vi "Test Data Acq.vi"() -> ()   [LabVIEW 2025]
doc: "Author: Scott Hannahs <sth@magnet.fsu.edu>\n\nThis software is licensed for use under the “MIT License\"\nCopyright (c) 2025 Scott Hannahs, sth@sth@magnet.sthnet.net\n\nPermission is hereby granted, free of charge, to any person obtaining a copy of this software and associated documentation files (the \"Software\"), to deal in the Software without restriction, including without limitation the rights to use, copy, modify, merge, publish, distribute, sublicense, and/or sell copies of the Software, and to permit persons to whom the Software is furnished to do so, subject to the following conditions: The above copyright notice and this permission notice shall be included in all copies or substantial portions of the Software.\n\nTHE SOFTWARE IS PROVIDED \"AS IS\", WITHOUT WARRANTY OF ANY KIND, EXPRESS OR IMPLIED, INCLUDING BUT NOT LIMITED TO THE WARRANTIES OF MERCHANTABILITY, FITNESS FOR A PARTICULAR PURPOSE AND NONINFRINGEMENT. IN NO EVENT SHALL THE AUTHORS OR COPYRIGHT HOLDERS BE LIABLE FOR ANY CLAIM, DAMAGES OR OTHER LIABILITY, WHETHER IN AN ACTION OF CONTRACT, TORT OR OTHERWISE, ARISING FROM, OUT OF OR IN CONNECTION WITH THE SOFTWARE OR THE USE OR OTHER DEALINGS IN THE SOFTWARE."
uses:
  Sub Controls/All Data Array.ctl
  Sub Controls/Instrument Properties.ctl
  Sub Controls/Public.ctl
  Sub Controls/Private.ctl
  Sub Controls/Instrument Ref.ctl
  Sub Controls/SystemCheckBox-resize.ctl
  Sub Controls/DataAcq User Events.ctl
panel:
  in  "New/Stop":bool
  out "All Data":T1 format="%^_6g"
  out "Labels":string[](array[string])=["Field", "Timestamp"]
  out "Data":dbl[](array[numeric])=[1.0, 0.02, 0.0, 0.0] format="%_4e"
  out "Colors":u32[](array[colorbox])=[16748168, 2796287]
  in  "Quit":bool
  in  "Test":bool
  in  "Configure":bool
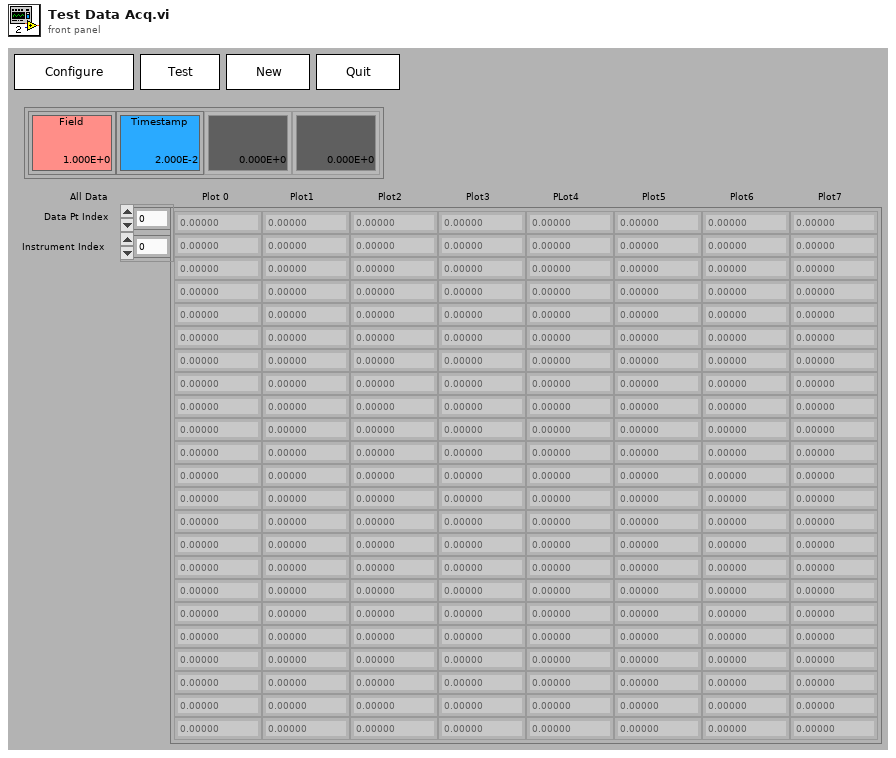
[diagram p1: front panel]
types:
  T1 = typedef "All Data Array.ctl" = dbl[][]
  T2 = typedef "DataAcq User Events.ctl" = enum16{"Update Data Display", "Store Data"}
  T3 = typedef "Instrument Properties.ctl" = cluster{"Public":T4, "Private":T5}
  T4 = typedef "Public.ctl" = cluster{"Column Name":string[], "Trace Color":u32[]}
  T5 = typedef "Private.ctl" = cluster{"Path":path, "VI Refnum":T6, "Name":string, "# of Values":i32, "Scale Factors":dbl[], "Display":T7[], "Offset":dbl[]}
  T6 = typedef "Instrument Ref.ctl" = refnum<vi>
  T7 = typedef "SystemCheckBox-resize.ctl" = bool
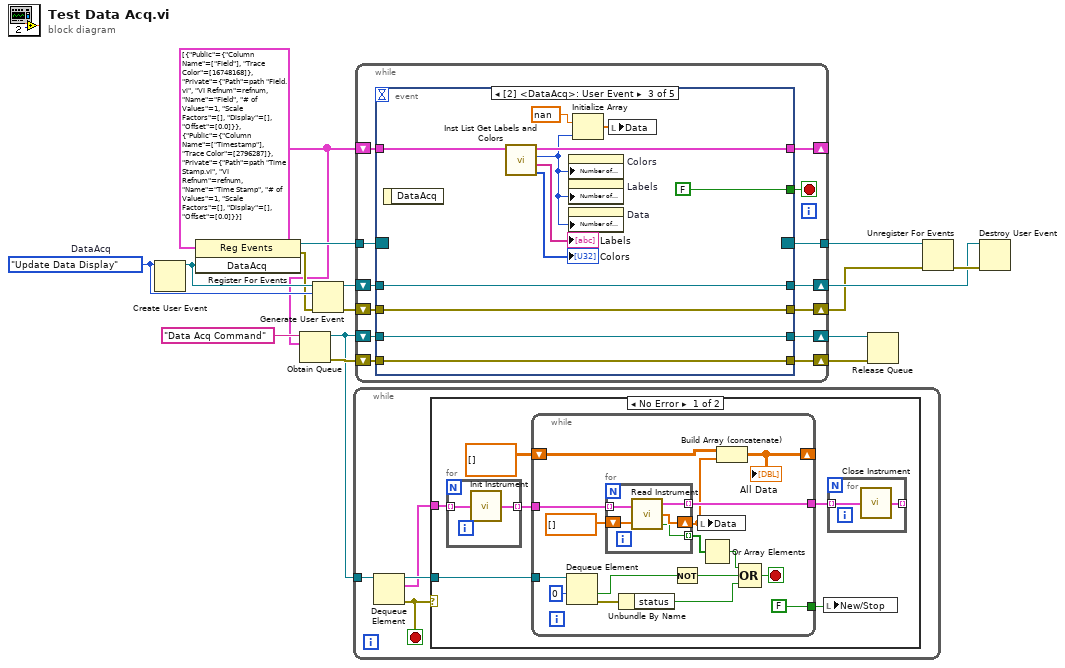
[diagram p0: block diagram]
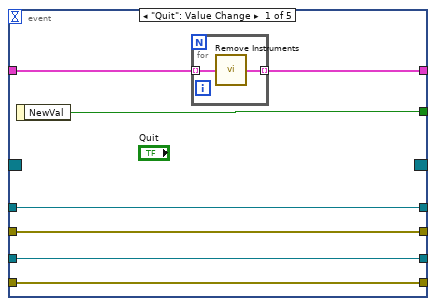
[diagram p3: hidden frame]
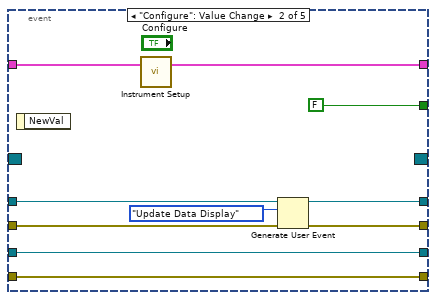
[diagram p4: hidden frame]
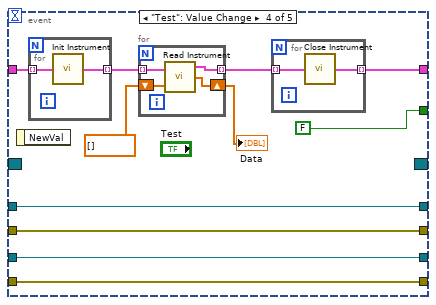
[diagram p5: hidden frame]
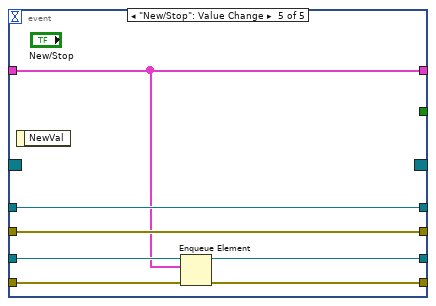
[diagram p6: hidden frame]
diagram:
  w14 = DataAcq_User_Events."Update Data Display"  # DataAcq
  w1 = T3[] [{"Public"={"Column Name"=["Field"], "Trace Color"=[16748168]}, "Private"={"Path"=path "Field.vi", "VI Refnum"=refnum, "Name"="Field", "# of Values"=1, "Scale Factors"=[], "Display"=[], "Offset"=[0.0]}}, {"Public"={"Column Name"=["Timestamp"], "Trace Color"=[2796287]}, "Private"={"Path"=path "Time Stamp.vi", "VI Refnum"=refnum, "Name"="Time Stamp", "# of Values"=1, "Scale Factors"=[], "Display"=[], "Offset"=[0.0]}}] ("Setup")
  n1 = Create User Event(user event datatype=w14) -> (user event=w15:refnum<user-event>)  [unwired: 1 in, 1 out]
  n2 = register-events(w15) -> (reference out=w16:refnum<event-registration>, error out=w13:errorcluster)  [unwired: 2 in]
  n3 = Obtain Queue(name (unnamed)="Data Acq Command", element data type=w1) -> (queue out=w3:refnum<queue>, error out=w5:errorcluster)  [unwired: 3 in, 1 out]
  n4 = Generate User Event(user event=w15, event data cluster=w14, error in=w13) -> (user event out=w12:refnum<user-event>, error out=w7:errorcluster)  [unwired: 1 in]
  n5 = while {
    tunnel: w3 -> [w20]
    stop <- w19 stop-if-true
    n6 = Dequeue Element(queue=w20) -> (queue out=w18:refnum<queue>, element=w17:T3[], error out=w19:errorcluster)  [unwired: 2 in, 1 out]
    n7 = case shown="No Error" w19 {
      tunnel: w18 -> [w22 _]
      tunnel: w17 -> [w26 _]
      frame No Error {
        n8 = for {
          tunnel: w26 -> [w51] mode=indexing
          tunnel: [w50] -> w25 mode=indexing
          n9 = call "Init Instrument.vi"("Instrument Prop"=w51) -> ("Instrument Prop 2"=w50:T3)
        }
        n10 = while {
          tunnel: w25 -> [w43]
          tunnel: [w42] -> w24
          shift-right: [w38] -> _
          shift-left: dbl[][] [] ("Array 2") -> [w37]
          tunnel: w22 -> [w34]
          tunnel: [FALSE ("New/Stop")] -> w21
          stop <- w39 stop-if-true
          n11 = Dequeue Element(queue=w34, timeout in ms (-1)=0) -> (timed out?=w35:bool, error out=w31:errorcluster)  [unwired: 1 in, 2 out]
          n12 = for {
            tunnel: w43 -> [w49] mode=indexing
            tunnel: [w48] -> w42 mode=indexing
            shift-right: [w46] -> w36
            shift-left: dbl[] [] ("Array 2") -> [w47]
            tunnel: [w45] -> w41 mode=indexing
            n13 = call "Read Instrument.vi"("Instrument Prop In"=w49, "Array In"=w47) -> ("Instrument Prop Out"=w48:T3, "Array Out"=w46:dbl[], "Stop"=w45:bool)
          }
          n14 = Unbundle By Name(w31) -> ("status"=w32:bool)
          n15 = Not(x=w35) -> (.not. x?=w30:bool)
          n16 = local write "Data"(w36) -> ()
          n17 = Or Array Elements(Boolean array=w41) -> (logical OR=w40:bool)
          n18 = Build Array (concatenate)(w37, w36) -> (w38:dbl[][])
          "All Data" <- w38
          n19 = Compound Arithmetic op=OR(w40, w30, w32) -> (w39:bool)
        }
        n20 = local write "New/Stop"(w21) -> ()
        n21 = for {
          tunnel: w24 -> [w28] mode=indexing
          tunnel: [w27] -> _ mode=indexing
          n22 = call "Close Instrument.vi"("Instrument Prop"=w28) -> ("Instrument Prop 2"=w27:T3)
        }
      }
      frame Error {
      }
    }
  }
  n23 = while {
    shift-right: [w63] -> _
    shift-left: w1 -> [w62]
    tunnel: w16 -> [w61]
    shift-right: [w59] -> w9
    shift-left: w12 -> [w60]
    tunnel: [w58] -> w11
    shift-right: [w56] -> w8
    shift-left: w3 -> [w57]
    shift-right: [w54] -> w6
    shift-left: w7 -> [w55]
    shift-right: [w52] -> w4
    shift-left: w5 -> [w53]
    stop <- w64 stop-if-true
    n24 = event shown="[2] <DataAcq>: User Event" {
      selector: w61 -> [_ _ _ _ _]
      dyn-events: [_ _ _ _ _] -> w58
      timeout: _ -> [_ _ _ _ _]
      tunnel: [w69 FALSE ("stop") FALSE ("stop") FALSE ("stop") _] -> w64
      tunnel: w62 -> [w71 w83 w93 w101 w115]
      tunnel: [w70 w78 w94 w99 w115] -> w63
      tunnel: w60 -> [w68 w81 w90 w103 w121]
      tunnel: [w68 w79 w90 w103 w121] -> w59
      tunnel: [w66 w75 w85 w98 w119] -> w56
      tunnel: w57 -> [w66 w75 w85 w98 w116]
      tunnel: [w67 w77 w86 w97 w120] -> w54
      tunnel: w55 -> [w67 w76 w86 w97 w120]
      tunnel: [w65 w74 w84 w96 w118] -> w52
      tunnel: w53 -> [w65 w74 w84 w96 w117]
      event "Quit": Value Change {
        n25 = event-data() -> ("NewVal"=w69:bool)  [unwired: 1 in]
        n26 = for {
          tunnel: w71 -> [w73] mode=indexing
          tunnel: [w72] -> w70 mode=indexing
          n27 = call "Remove Instruments.vi"("Instrument Prop"=w73) -> ("Instrument Prop Out"=w72:T3)
        }
      }
      event "Configure": Value Change {
        n28 = event-data() -> ()  [unwired: 1 in, 1 out]
        n29 = call "Instrument Setup.vi"("Configured Inst"=w83) -> ("Configured Inst dup"=w78:T3[])  [unwired: 2 in]
        n30 = Generate User Event(user event=w81, event data cluster=DataAcq_User_Events."Update Data Display" ("event data"), error in=w76) -> (user event out=w79:refnum<user-event>, error out=w77:errorcluster)  [unwired: 1 in]
      }
      event User Event {
        n31 = event-data() -> ()  [unwired: 1 in, 1 out]
        n32 = call "Inst List Get Labels and Colors.vi"("Instrument List"=w93) -> ("Colors"=→"Colors":u32[], "Labels"=→"Labels":string[], "Number of Columns"=w87:u32, "Instrument List Out"=w94:T3[])  [unwired: 4 in, 3 out]
        n33 = property on="Colors" class="Arr (strict)"("Number of Columns"=w87) -> ()  [unwired: 2 in, 2 out]
        n34 = property on="Labels" class="Arr (strict)"("Number of Columns"=w87) -> ()  [unwired: 2 in, 2 out]
        n35 = property on="Data" class="Arr (strict)"("Number of Columns"=w87) -> ()  [unwired: 2 in, 2 out]
        n36 = Initialize Array(nan, w87) -> (w89:dbl[])
        n37 = local write "Data"(w89) -> ()
      }
      event "Test": Value Change {
        n38 = event-data() -> ()  [unwired: 1 in, 1 out]
        n39 = for {
          tunnel: w101 -> [w110] mode=indexing
          tunnel: [w109] -> w102 mode=indexing
          n40 = call "Init Instrument.vi"("Instrument Prop"=w110) -> ("Instrument Prop 2"=w109:T3)
        }
        n41 = for {
          tunnel: w102 -> [w114] mode=indexing
          tunnel: [w113] -> w100 mode=indexing
          shift-right: [w111] -> w104
          shift-left: dbl[] [] ("Array 2") -> [w112]
          n42 = call "Read Instrument.vi"("Instrument Prop In"=w114, "Array In"=w112) -> ("Instrument Prop Out"=w113:T3, "Array Out"=w111:dbl[])  [unwired: 1 out]
        }
        "Data" <- w104
        n43 = for {
          tunnel: w100 -> [w108] mode=indexing
          tunnel: [w107] -> w99 mode=indexing
          n44 = call "Close Instrument.vi"("Instrument Prop"=w108) -> ("Instrument Prop 2"=w107:T3)
        }
      }
      event "New/Stop": Value Change {
        n45 = event-data() -> ()  [unwired: 1 in, 1 out]
        n46 = Enqueue Element(queue=w116, element=w115, error in (no error)=w117) -> (queue out=w119:refnum<queue>, error out=w118:errorcluster)  [unwired: 1 in, 1 out]
      }
    }
  }
  n47 = Release Queue(queue=w8, error in (no error)=w4) -> ()  [unwired: 1 in, 3 out]
  n48 = Unregister For Events(event registration refnum=w11, error in=w6) -> (error out=w10:errorcluster)
  n49 = Destroy User Event(user event=w9, error in=w10) -> ()  [unwired: 1 out]
